vi "NiFPGA Read Array - I16.vi"(7 "Size":u32, 8 "error in (no error)":errorcluster, 10 "Indicator":u32, 11 "Session":u32) -> (0 "error out":errorcluster, 1 "Array":i16[](array[numeric]), 3 "Session Out":u32)   [LabVIEW 2010, in "FPGA Interface Wrapper.lvlib"]
doc: "Reads an entire array of signed 16-bit integer values from a given array indicator or control."
uses:
  <userlib>/_FPGA Interface Advanced Tools/FPGA Interface Wrapper/FPGA Interface Wrapper.lvlib
  NiFpga.dll
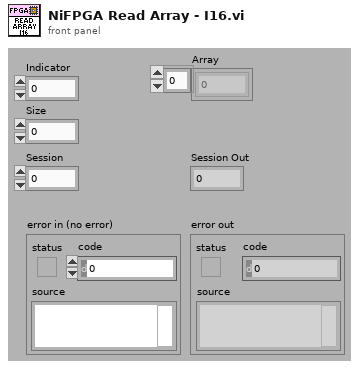
[diagram p1: front panel]
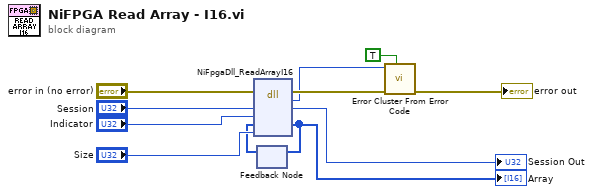
[diagram p0: block diagram]
diagram:
  n1 = feedback #1() -> (w4:i16[])  [unwired: 1 in]
  n2 = dll-call lib="NiFpga.dll" fn="NiFpgaDll_ReadArrayI16"(error in="error in (no error)", "Session"="Session", "Indicator"="Indicator", "Array"=w4, "Size"="Size") -> (error out=w2:errorcluster, "Status"=w1:i32, "Session"=→"Session Out":u32, "Array"=w5:i16[])  [unwired: 4 in, 1 out]
  "Array" <- w5
  n3 = feedback-in #1(w5) -> ()
  n4 = call <vilib>:"Error Cluster From Error Code.vi"("show call chain? (False)"=TRUE, "error in (no error)"=w2, "error code (0)"=w1) -> ("error out"=→"error out":errorcluster)  [unwired: 6 in]
